vi "_시리얼-패킷 데이타-수신 - GEN4 1st PP.vi"(6 "ErrIn":bool, 7 "시리얼 포트":refnum<visa-resource-name>="COM9") -> (0 "수신 문자열 버퍼":string, 1 "수신 문자열":string, 2 "Processing TIme(ms)":u32=1, 3 "수신 실패(T)":bool)   [LabVIEW 2015]
panel:
  out "재시도":i32
  out "정상패킷 검출":bool
  out "웨이브폼 차트":u32(graph)=1
  out "에러 출력":errorcluster={"status"=FALSE, "code"=1073676294, "source"="_시리얼-패킷 데이타-수신.vi 안에 VISA 읽기"}
  out "수신 타이머 값":u32=5982350
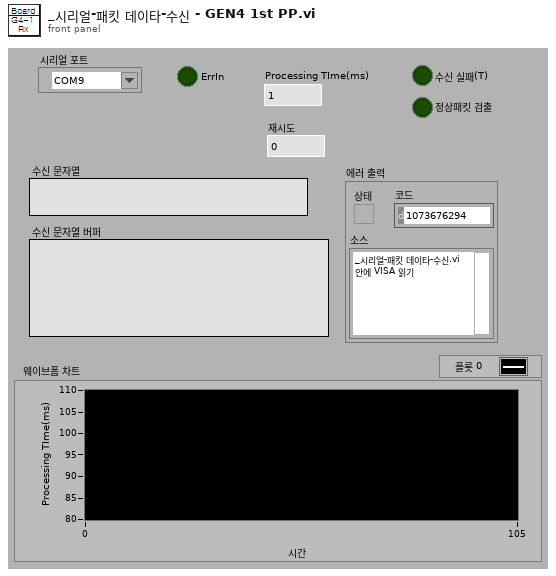
[diagram p1: front panel]
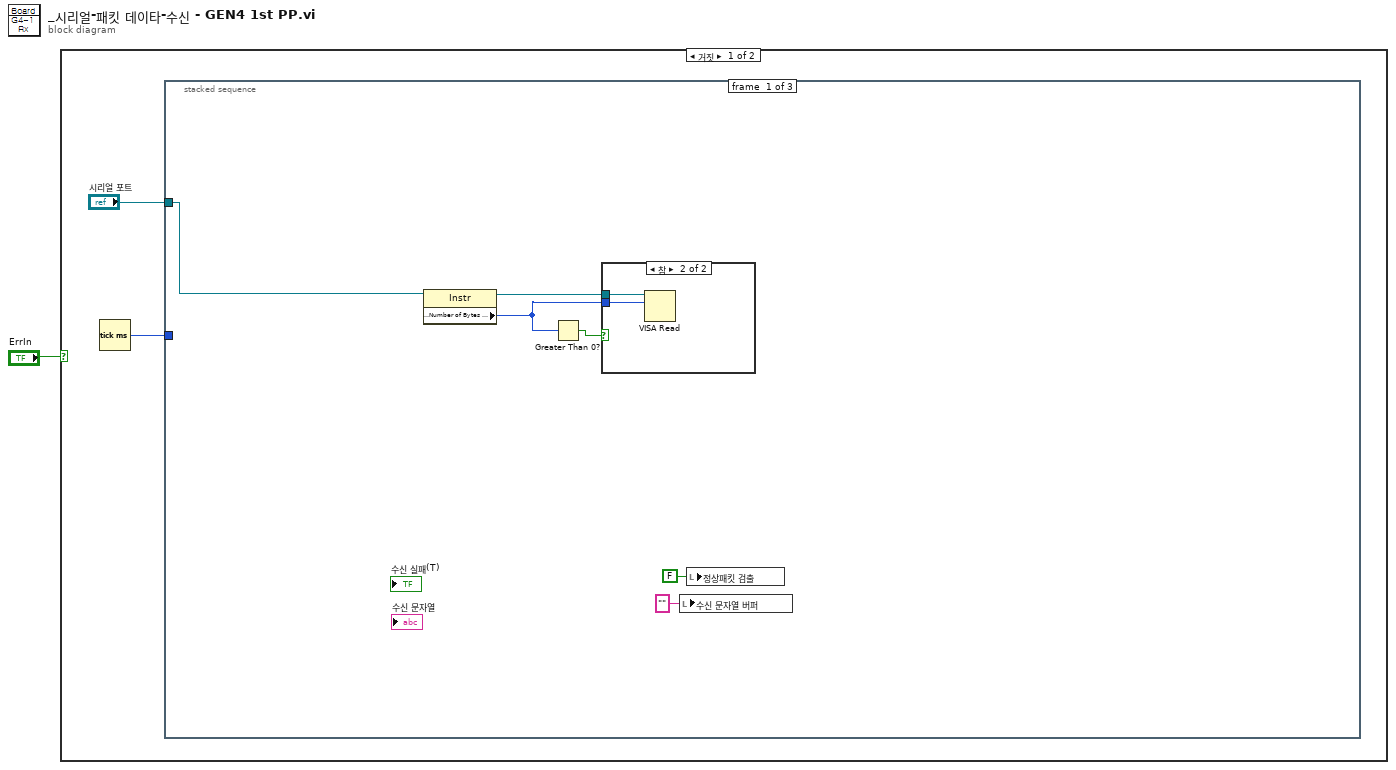
[diagram p0: block diagram]
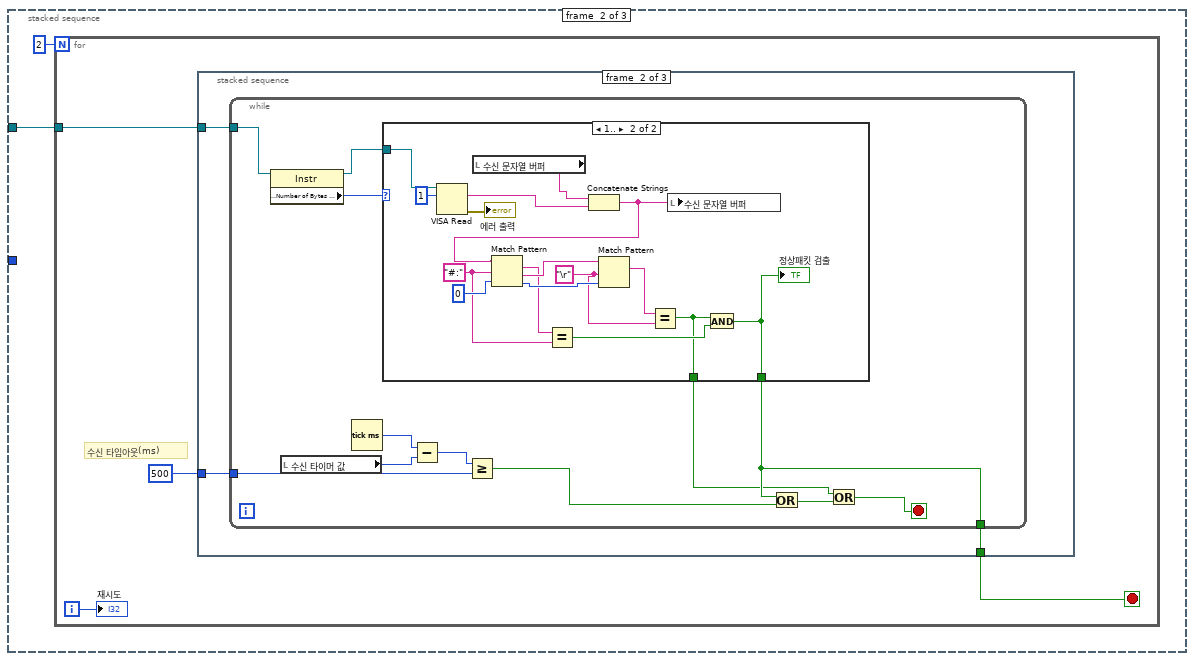
[diagram p3: hidden frame]
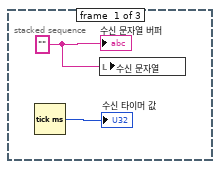
[diagram p4: hidden frame]
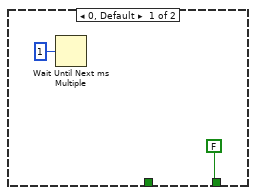
[diagram p5: hidden frame]
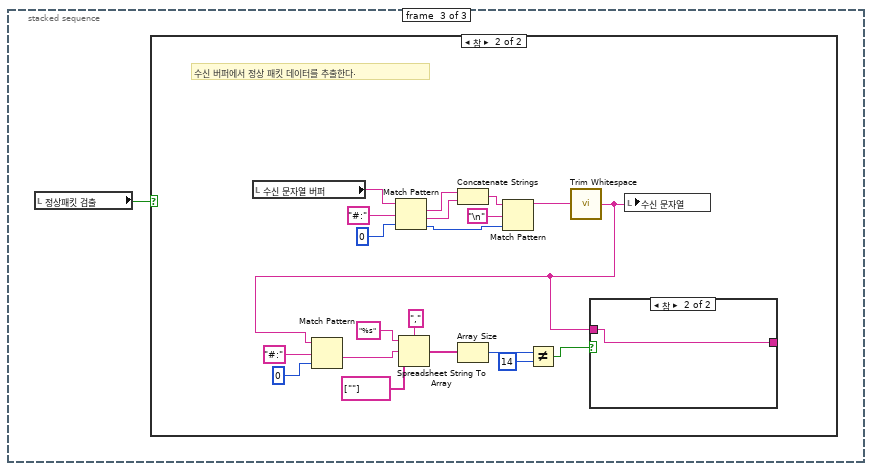
[diagram p6: hidden frame]
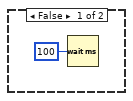
[diagram p7: hidden frame]
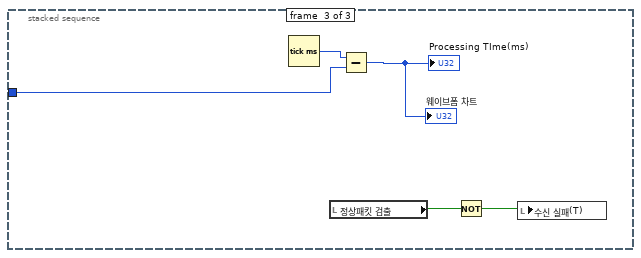
[diagram p9: hidden frame]
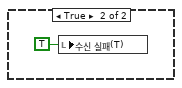
[diagram p10: hidden frame]
diagram:
  n1 = case shown="거짓" "ErrIn" {
    frame False {
      n2 = Tick Count (ms)() -> (millisecond timer value=w2:u32)
      n3 = stacked-sequence {
        tunnel: "시리얼 포트" -> [w9 w13 _]
        tunnel: w2 -> [_ _ w79]
        frame #0 {
          n4 = property class="Instr"(reference=w9) -> (reference out=w6:refnum<visa-resource-name>, "Serial Settings:Number of Bytes at Serial Port"=w5:u32)  [unwired: 1 in, 1 out]
          n5 = Greater Than 0?(x=w5) -> (x > 0?=w4:bool)
          n6 = case shown="참" w4 {
            tunnel: w6 -> [_ w11]
            tunnel: w5 -> [_ w10]
            frame False {
            }
            frame True {
              n7 = VISA Read(VISA resource name=w11, byte count=w10) -> ()  [unwired: 1 in, 4 out]
            }
          }
          n8 = local write "수신 문자열 버퍼"("" ("수신 문자열 버퍼")) -> ()
          n9 = local write "정상패킷 검출"(FALSE ("정상패킷 검출")) -> ()
        }
        frame #1 {
          n10 = for {
            N: 2 -> [_]
            tunnel: w13 -> [w16]
            i -> [w14]
            stop <- w15 stop-if-true
            # "수신 타임아웃(ms)"
            n11 = stacked-sequence {
              tunnel: w16 -> [_ w22 _]
              tunnel: 500 -> [_ w21 _]
              tunnel: [_ w20 _] -> w15
              frame #0 {
                w18 = "" ("수신 문자열")
                n12 = Tick Count (ms)() -> (millisecond timer value=→"수신 타이머 값":u32)
                n13 = local write "수신 문자열"(w18) -> ()
                "수신 문자열 버퍼" <- w18
              }
              frame #1 {
                n14 = while {
                  tunnel: w22 -> [w34]
                  tunnel: w21 -> [w30]
                  tunnel: [w26] -> w20
                  stop <- w23 stop-if-true
                  n15 = property class="Instr"(reference=w34) -> (reference out=w27:refnum<visa-resource-name>, "Serial Settings:Number of Bytes at Serial Port"=w29:u32)  [unwired: 1 in, 1 out]
                  n16 = local read "수신 타이머 값"() -> (w32:u32)
                  n17 = Tick Count (ms)() -> (millisecond timer value=w33:u32)
                  n18 = case shown="1.." w29 {
                    tunnel: w27 -> [_ w51]
                    tunnel: [FALSE w40] -> w26
                    tunnel: [_ w38] -> w24
                    frame 0, Default {
                      n19 = Wait Until Next ms Multiple(millisecond multiple=u32 1 ("ms 배수")) -> ()  [unwired: 1 out]
                    }
                    frame 1.. {
                      w37 = "\r" ("검색 문자열")
                      w43 = "#:" ("검색 문자열")
                      n20 = VISA Read(VISA resource name=w51, byte count=u32 1 ("바이트 카운트")) -> (read buffer=w50:string, error out=→"에러 출력":errorcluster)  [unwired: 1 in, 2 out]
                      n21 = local read "수신 문자열 버퍼"() -> (w52:string)
                      n22 = Concatenate Strings(w52, w50) -> (w48:string)
                      n23 = Match Pattern(string=w48, regular expression=w43, offset (0)=0 ("오프셋(0)")) -> (match substring=w44:string, after substring=w46:string, offset past match=w45:i32)  [unwired: 1 out]
                      n24 = Equal?(x=w44, y=w43) -> (x = y?=w41:bool)
                      n25 = Match Pattern(string=w46, regular expression=w37, offset (0)=w45) -> (match substring=w42:string)  [unwired: 3 out]
                      n26 = Equal?(x=w42, y=w37) -> (x = y?=w38:bool)
                      n27 = local write "수신 문자열 버퍼"(w48) -> ()
                      n28 = And(x=w38, y=w41) -> (x .and. y?=w40:bool)
                      "정상패킷 검출" <- w40
                    }
                  }
                  n29 = Subtract(x=w33, y=w32) -> (x-y=w31:u32)
                  n30 = Greater Or Equal?(x=w31, y=w30) -> (x >= y?=w28:bool)
                  n31 = Or(x=w26, y=w28) -> (x .or. y?=w25:bool)
                  n32 = Or(x=w24, y=w25) -> (x .or. y?=w23:bool)
                }
              }
              frame #2 {
                n33 = local read "정상패킷 검출"() -> (w53:bool)
                n34 = case shown="참" w53 {
                  frame False {
                    n35 = Wait (ms)(milliseconds to wait=u32 100 ("대기 시간(ms)")) -> ()  [unwired: 1 out]
                  }
                  frame True {
                    # "수신 버퍼에서 정상 패킷 데이터를 추출한다."
                    n36 = local read "수신 문자열 버퍼"() -> (w70:string)
                    n37 = Match Pattern(string=w70, regular expression="#:" ("검색 문자열"), offset (0)=0 ("오프셋(0)")) -> (match substring=w67:string, after substring=w66:string, offset past match=w73:i32)  [unwired: 1 out]
                    n38 = Concatenate Strings(w67, w66) -> (w68:string)
                    n39 = Match Pattern(string=w68, regular expression="\n", offset (0)=w73) -> (before substring=w69:string)  [unwired: 3 out]
                    n40 = call <vilib>:"Trim Whitespace.vi"("string"=w69) -> ("trimmed string"=w55:string)  [unwired: 1 in]
                    n41 = Match Pattern(string=w55, regular expression="#:" ("검색 문자열"), offset (0)=0 ("오프셋(0)")) -> (after substring=w60:string)  [unwired: 3 out]
                    n42 = Spreadsheet String To Array(delimiter (Tab)="," ("구분 문자(탭)"), format string="%s" ("스프레드시트 문자열"), spreadsheet string=w60, array type (2D Dbl)=string[] [""] ("배열 타입(2D Dbl)")) -> (array=w59:string[])
                    n43 = Array Size(array=w59) -> (size(s)=w58:i32)
                    n44 = Not Equal?(x=w58, y=14) -> (x != y?=w56:bool)
                    n45 = case shown="참" w56 {
                      tunnel: w55 -> [_ w75]
                      tunnel: [_ w75] -> _
                      frame False {
                      }
                      frame True {
                      }
                    }
                    n46 = local write "수신 문자열"(w55) -> ()
                  }
                }
              }
            }
            "재시도" <- w14
          }
        }
        frame #2 {
          n47 = Tick Count (ms)() -> (millisecond timer value=w80:u32)
          n48 = local read "정상패킷 검출"() -> (w77:bool)
          n49 = Subtract(x=w80, y=w79) -> (x-y=→"Processing TIme(ms)" →"웨이브폼 차트":u32)
          n50 = Not(x=w77) -> (.not. x?=w76:bool)
          n51 = local write "수신 실패(T)"(w76) -> ()
        }
      }
    }
    frame True {
      n52 = local write "수신 실패(T)"(TRUE ("수신 실패(T)")) -> ()
    }
  }
